vi "sub_motion.vi"(10 "vy":cluster{"v":dbl, "u":dbl}, 11 "x":dbl[](array[numeric])) -> (3 "x out":dbl[](array[numeric]))   [LabVIEW 2019]
uses:
  Ctrl/cmd_common.ctl
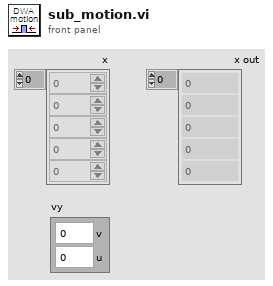
[diagram p1: front panel]
types:
  T1 = typedef "cmd_common.ctl" = enum16{"read", "write"}
  T2 = cluster{"x":dbl[], "dw":dbl[], "vy":cluster{"v":dbl, "y":dbl}, "trajectory":dbl[][], "best trajectory":dbl[][], "best u":cluster{"v":dbl, "y":dbl}}
  T3 = cluster{"max speed":dbl, "min speed":dbl, "max yaw rate":dbl, "max accel":dbl, "max delta yaw rate":dbl, "v resolution":dbl, "yaw rate resolution":dbl, "dt":dbl, "predict time":dbl, "to goal cost gain":dbl, "speed cost gain":dbl, "obstacle cost gain":dbl, "robot stuck flag cons":dbl, "robot type":enum16{"circle", "rectangle"}, "robot radius":dbl, "robot width":dbl, "robot length":dbl, "obstacles":cluster{"x":dbl, "y":dbl}[], "goal pt":cluster{"x":i32, "y":i32}}
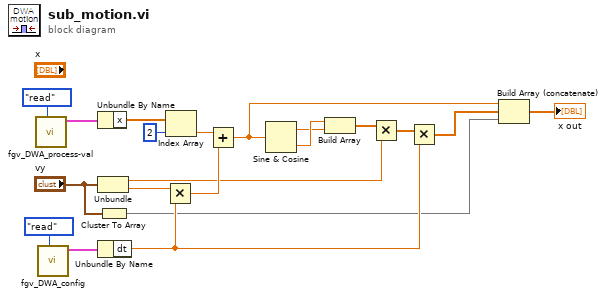
[diagram p0: block diagram]
diagram:
  n1 = call "fgv_DWA_process-val.vi"("cmd"=cmd_common."read") -> ("prcess val out"=w19:T2)  [unwired: 10 in]
  n2 = call "fgv_DWA_config.vi"("cmd"=cmd_common."read") -> ("config out"=w16:T3)  [unwired: 10 in]
  n3 = Unbundle By Name(w19) -> ("x"=w18:dbl[])
  n4 = Unbundle("vy") -> ("v"=w10:dbl, "u"=w14:dbl)
  n5 = Unbundle By Name(w16) -> ("dt"=w8:dbl)
  n6 = Cluster To Array(cluster="vy") -> (array=w3:dbl[])
  n7 = Multiply(x=w14, y=w8) -> (x*y=w13:dbl)
  n8 = Index Array(array=w18, index=2) -> (element=w15:dbl)
  n9 = Add(x=w15, y=w13) -> (x+y=w4:dbl)
  n10 = Sine & Cosine(0:w4) -> (1:w6:dbl, 2:w7:dbl)
  n11 = Build Array(w7, w6) -> (w11:dbl[])
  n12 = Multiply(x=w11, y=w10) -> (x*y=w9:dbl[])
  n13 = Multiply(x=w9, y=w8) -> (x*y=w5:dbl[])
  n14 = Build Array (concatenate)(w4, w5, w3) -> (→"x out":dbl[])
